vi "AK-Seriell FGV.vi"(6 "Aktionen":T2, 8 "error in":errorcluster caption="error out", 10 "Serielle Parameter":T1={"VISA resource name"="COM1", "baud rate"=38400, "data bits"=8, "parity"=0, "stop bits"=10, "flow control"=0} {"flow control" items=["None"=0, "XON/XOFF"=1, "RTS/CTS"=2, "DTR/DSR"=4]; "stop bits" items=["1.0"=10, "1.5"=15, "2.0"=20]; "parity" items=["None", "Odd", "Even", "Mark", "Space"]; "data bits" min=5 max=8 step=1}) -> (0 "error out":errorcluster, 2 "Serielle Parameter 2":T1={"VISA resource name"="COM1", "baud rate"=38400, "data bits"=8, "parity"=0, "stop bits"=10, "flow control"=0} {"flow control" items=["None"=0, "XON/XOFF"=1, "RTS/CTS"=2, "DTR/DSR"=4]; "stop bits" items=["1.0"=10, "1.5"=15, "2.0"=20]; "parity" items=["None", "Odd", "Even", "Mark", "Space"]; "data bits" min=5 max=8 step=1})   [LabVIEW 2020, in "AK-Schnittstelle.lvlib" / "AK Seriell.lvlib"]
uses:
  AK Seriell/AK Seriell.lvlib
  Aktionen AK.ctl
  Serielle Parameter.ctl
  Daten weitergeben Aktionen.ctl
  Aktionen Gespeicherte Werte.ctl
  <vilib>/Instr/_visa.llb/VISA Configure Serial Port (Instr).vi
  AK-Schnittstelle.lvlib
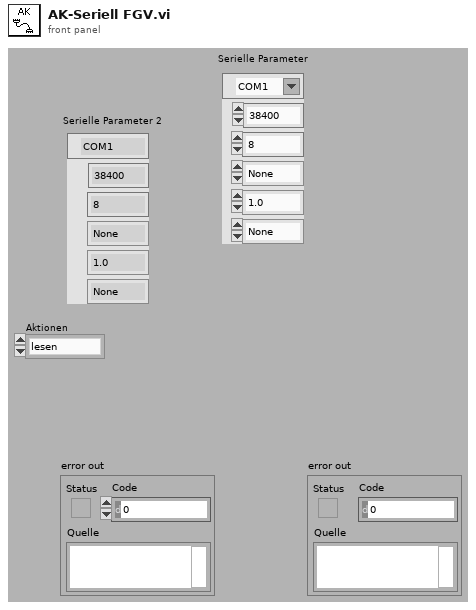
[diagram p1: front panel]
types:
  T1 = typedef "AK-Schnittstelle.lvlib/AK Seriell.lvlib/Serielle Parameter.ctl" = cluster{"VISA resource name":refnum<visa-resource-name>, "baud rate":u32, "data bits":u16, "parity":u16, "stop bits":u16, "flow control":u16}
  T2 = typedef "AK-Schnittstelle.lvlib/Aktionen AK.ctl" = enum16{"lesen", "initialisieren", "beenden", "AK Komm"}
  T3 = typedef "AK-Schnittstelle.lvlib/Daten weitergeben Aktionen.ctl" = enum16{"lesen", "schreiben", "Log löschen", "Detail", "Detail löschen", "Speicher Freigeben"}
  T4 = typedef "AK-Schnittstelle.lvlib/Aktionen Gespeicherte Werte.ctl" = enum16{"lesen", "laden", "speichern", "Seriell", "TCP", "Diverse", "AKTIV", "AK-Namen"}
  T5 = typedef "AK-Schnittstelle.lvlib/Diverse gespeicherte Werte.ctl" = cluster{"Kalibriergaseingang":i16, "SamplePoint":i16, "CalGas zu PNS":i16, "Gas-Reihenfolge":i16[], "Zeit 0-Gas":sgl, "Zeit CalGas":sgl, "AK Befehlssatz":T6}
  T6 = typedef "AK-Schnittstelle.lvlib/AK Befehlssatz.ctl" = enum16{"MEXA", "IAG v1.4", "AVL (Puma)", "PEUS"}
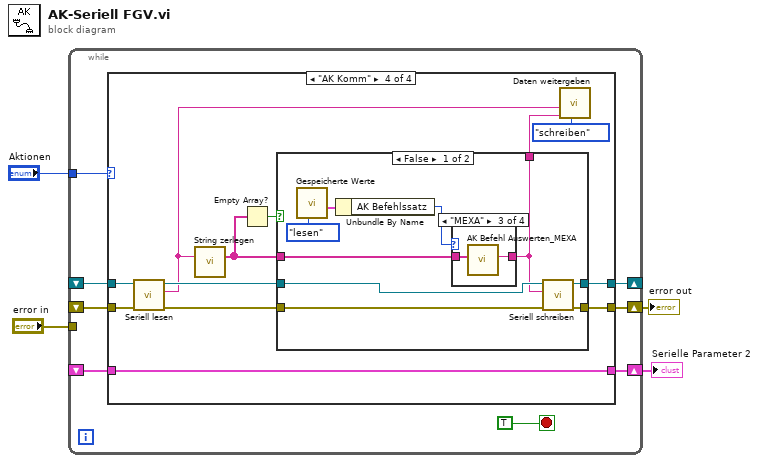
[diagram p0: block diagram]
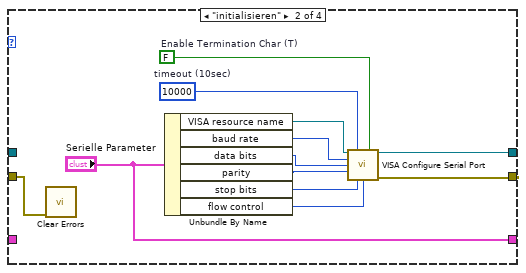
[diagram p3: hidden frame]
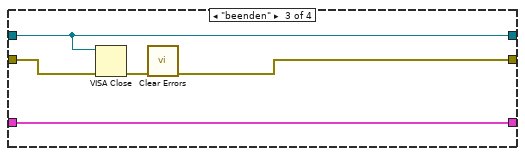
[diagram p4: hidden frame]
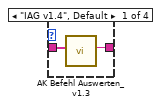
[diagram p5: hidden frame]
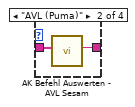
[diagram p6: hidden frame]
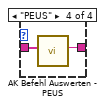
[diagram p7: hidden frame]
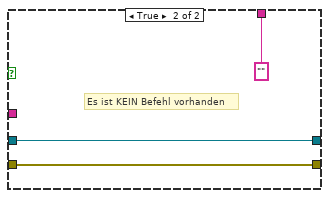
[diagram p8: hidden frame]
diagram:
  n1 = while {
    tunnel: "Aktionen" -> [w11]
    shift-right: [w10] -> _
    shift-left: _ -> [w8]
    shift-right: [w9] -> w3
    shift-left: _ -> [w7]
    tunnel: "error in" -> [_]
    shift-right: [w6] -> w1
    shift-left: _ -> [w5]
    stop <- TRUE stop-if-true
    n2 = case shown="\"AK Komm\"" w11 {
      tunnel: [w15 w19 w31 w44] -> w10
      tunnel: [w14 w18 w29 w43] -> w9
      tunnel: w8 -> [w15 _ w31 w42]
      tunnel: w7 -> [w14 w17 w32 w34]
      tunnel: [w13 "Serielle Parameter" w28 w33] -> w6
      tunnel: w5 -> [w13 _ w28 w33]
      frame "lesen", Default {
      }
      frame "initialisieren" {
        w27 = FALSE  # Enable Termination Char (T)
        w26 = u32 10000  # timeout (10sec)
        n3 = call <vilib>:"Clear Errors.vi"("error in (no error)"=w17) -> ()  [unwired: 5 in, 2 out]
        n4 = Unbundle By Name("Serielle Parameter") -> ("VISA resource name"=w25:refnum<visa-resource-name>, "baud rate"=w24:u32, "data bits"=w23:u16, "parity"=w22:u16, "stop bits"=w21:u16, "flow control"=w20:u16)
        n5 = call-poly "VISA Configure Serial Port"("VISA resource name"=w25, "timeout (10sec)"=w26, "Enable Termination\nChar (T)"=w27, "baud rate (9600)"=w24, "data bits (8)"=w23, "parity (0:none)"=w22, "stop bits (10: 1 bit)"=w21, "flow control (0:none)"=w20) -> ("VISA resource name out"=w19:refnum<visa-resource-name>, "error out"=w18:errorcluster)  [unwired: 1 in, 5 out]
      }
      frame "beenden" {
        n6 = VISA Close(VISA resource name=w31, error in (no error)=w32) -> (error out=w30:errorcluster)
        n7 = call <vilib>:"Clear Errors.vi"("error in (no error)"=w30) -> ("error out"=w29:errorcluster)  [unwired: 5 in, 1 out]
      }
      frame "AK Komm" {
        n8 = call "Seriell lesen.vi"("Fehler (Eingang)"=w34, "VISA resource name"=w42) -> ("error out"=w39:errorcluster, "read buffer"=w36:string, "VISA resource name"=w41:refnum<visa-resource-name>)  [unwired: 6 in, 1 out]
        n9 = call "String zerlegen.vi"("read buffer"=w36) -> ("Array"=w38:string[])  [unwired: 14 in]
        n10 = Empty Array?(array=w38) -> (empty?=w40:bool)
        n11 = case shown="False" w40 {
          tunnel: [w53 w64] -> w44
          tunnel: [w52 w63] -> w43
          tunnel: w38 -> [w49 _]
          tunnel: w41 -> [w51 w64]
          tunnel: w39 -> [w45 w63]
          tunnel: [w48 "" ("String für schreiben")] -> w35
          frame False {
            n12 = call "Gespeicherte Werte.vi"("Aktionen"=Aktionen_Gespeicherte_Werte."lesen") -> ("Diverse Werte"=w47:T5)  [unwired: 6 in, 4 out]
            n13 = Unbundle By Name(w47) -> ("AK Befehlssatz"=w46:T6)
            n14 = case shown="\"MEXA\"" w46 {
              tunnel: w49 -> [w55 w57 w59 w60]
              tunnel: [w54 w56 w58 w61] -> w48
              frame "IAG v1.4", Default {
                n15 = call "AK Befehl Auswerten_v1.3.vi"("Array"=w55) -> ("String für schreiben"=w54:string)  [unwired: 10 in]
              }
              frame "AVL (Puma)" {
                n16 = call "AK Befehl Auswerten - AVL Sesam.vi"("Array"=w57) -> ("String für schreiben"=w56:string)  [unwired: 10 in]
              }
              frame "MEXA" {
                n17 = call "AK Befehl Auswerten_MEXA.vi"("Array"=w59) -> ("String für schreiben"=w58:string)  [unwired: 10 in]
              }
              frame "PEUS" {
                n18 = call "AK Befehl Auswerten - PEUS.vi"("Array"=w60) -> ("String für schreiben"=w61:string)  [unwired: 10 in]
              }
            }
            n19 = call "Seriell schreiben.vi"("error in"=w45, "String"=w48, "VISA resource name"=w51) -> ("error out 2"=w52:errorcluster, "VISA resource name"=w53:refnum<visa-resource-name>)  [unwired: 6 in, 1 out]
          }
          frame True {
            # "Es ist KEIN Befehl vorhanden"
          }
        }
        n20 = call "Daten weitergeben.vi"("Aktionen"=Daten_weitergeben_Aktionen."schreiben", "Antwort"=w35, "Empfangspuffer"=w36) -> ()  [unwired: 4 in, 5 out]
      }
    }
  }
  "error out" <- w3
  "Serielle Parameter 2" <- w1
